vi "SHA-1_for_text_file.vi"(8 "error in (no error)":errorcluster, 11 "text file path (use dialog)":path) -> (0 "error out":errorcluster, 3 "hash":string)   [LabVIEW 2015]
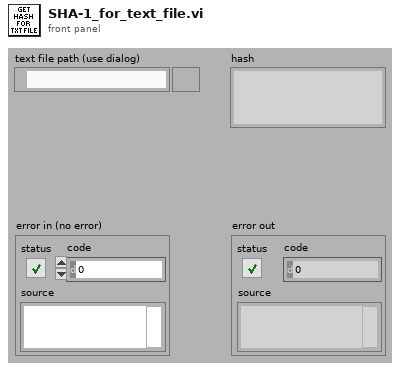
[diagram p1: front panel]
types:
  T1 = enum16{"open", "replace", "create", "open or create", "replace or create", "replace or create with confirmation"}
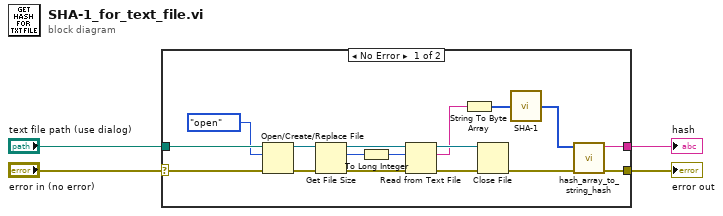
[diagram p0: block diagram]
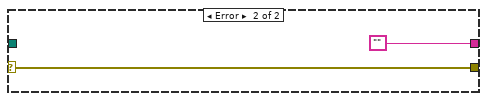
[diagram p2: hidden frame]
diagram:
  n1 = case shown="No Error" "error in (no error)" {
    selector: "error in (no error)" -> [w14 w23]
    tunnel: [w6 w23] -> w4
    tunnel: "text file path (use dialog)" -> [w18 _]
    tunnel: [w5 ""] -> w1
    frame No Error {
      n2 = Open/Create/Replace File(file path (use dialog)=w18, error in=w14, operation (0:open)=T1."open") -> (refnum out=w16:refnum<file>, error out=w21:errorcluster)  [unwired: 3 in, 1 out]
      n3 = Get File Size(file=w16, error in=w21) -> (refnum out=w11:refnum<file>, size (in bytes)=w15:i64, 0:w20:errorcluster)
      n4 = To Long Integer(number=w15) -> (32bit integer=w12:i32)
      n5 = Read from Text File(file (use dialog)=w11, count=w12, error in=w20) -> (refnum out=w13:refnum<file>, text=w10:string, error out=w19:errorcluster)  [unwired: 1 in, 1 out]
      n6 = String To Byte Array(string=w10) -> (unsigned byte array=w9:u8[])
      n7 = Close File(refnum=w13, error in=w19) -> (error out=w7:errorcluster)  [unwired: 1 out]
      n8 = call "SHA-1.vi"("Data"=w9) -> ("message-digest"=w8:u8[])
      n9 = call "hash_array_to_string_hash.vi"("error in (no error)"=w7, "message-digest"=w8) -> ("error out"=w6:errorcluster, "result string"=w5:string)  [unwired: 8 in]
    }
    frame Error {
    }
  }
  "error out" <- w4
  "hash" <- w1
